vi "Save-Screen-Shot.vi"(11 "VI Path":path) -> (0 "error out":errorcluster)   [LabVIEW 2017]
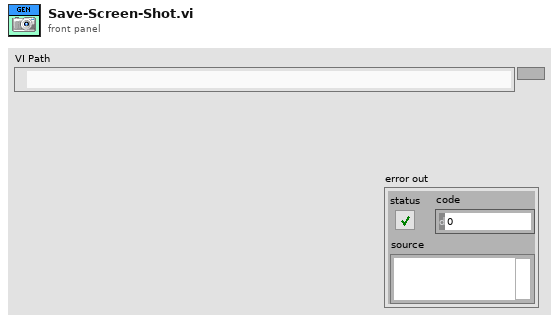
[diagram p1: front panel]
types:
  T1 = typedef "imagedata.ctl" = cluster{"image type":i32, "image depth":i32, "image":u8[], "mask":u8[], "colors":u32[], "Rectangle":cluster{"left":i16, "top":i16, "right":i16, "bottom":i16}}
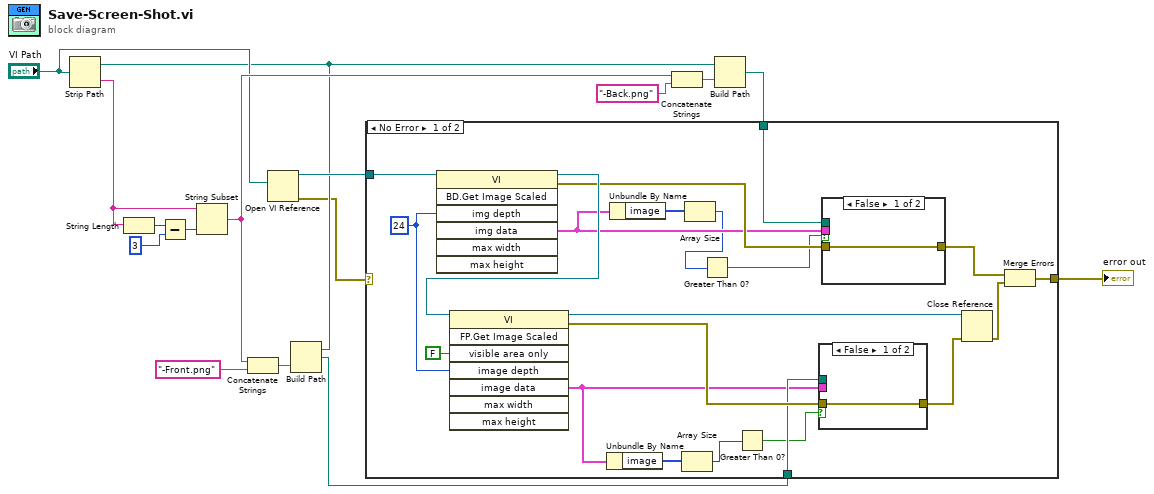
[diagram p0: block diagram]
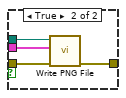
[diagram p2: hidden frame]
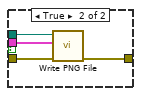
[diagram p3: hidden frame]
diagram:
  n1 = Strip Path(path="VI Path") -> (stripped path=w3:path, name=w2:string)
  n2 = String Length(string=w2) -> (length=w5:i32)
  n3 = Subtract(x=w5, y=3) -> (x-y=w7:i32)
  n4 = String Subset(string=w2, length (rest)=w7) -> (substring=w11:string)  [unwired: 1 in]
  n5 = Concatenate Strings(w11, "-Front.png" ("replace string (\"\")")) -> (w15:string)
  n6 = Open VI Reference(vi path="VI Path") -> (vi reference=w9:refnum<vi>, error out=w1:errorcluster)  [unwired: 5 in]
  n7 = Build Path(base path=w3, name or relative path=w15) -> (appended path=w14:path)
  n8 = Concatenate Strings(w11, "-Back.png" ("replace string (\"\")")) -> (w13:string)
  n9 = Build Path(base path=w3, name or relative path=w13) -> (appended path=w10:path)
  n10 = case shown="No Error" w1 {
    selector: w1 -> [_ w48]
    tunnel: [w33 w48] -> w16
    tunnel: w14 -> [w31 _]
    tunnel: w10 -> [w27 _]
    tunnel: w9 -> [w26 _]
    frame No Error {
      w29 = 24 ("Image Depth")
      n11 = invoke class="VI" method="BD.Get Image Scaled"(reference=w26, "img depth"=w29) -> (reference out=w28:refnum<vi>, error out=w25:errorcluster, "img data"=w24:T1)  [unwired: 5 in, 4 out]
      n12 = invoke class="VI" method="FP.Get Image Scaled"(reference=w28, "visible area only"=FALSE ("Visible Area Only"), "image depth"=w29) -> (reference out=w34:refnum<vi>, error out=w35:errorcluster, "image data"=w19:T1)  [unwired: 5 in, 5 out]
      n13 = Unbundle By Name(w19) -> ("image"=w20:u8[])
      n14 = Unbundle By Name(w24) -> ("image"=w23:u8[])
      n15 = Array Size(array=w20) -> (size(s)=w18:i32)
      n16 = Array Size(array=w23) -> (size(s)=w22:i32)
      n17 = Greater Than 0?(x=w22) -> (x > 0?=w21:bool)
      n18 = Greater Than 0?(x=w18) -> (x > 0?=w17:bool)
      n19 = case shown="False" w17 {
        tunnel: [w38 w42] -> w36
        tunnel: w35 -> [w38 w41]
        tunnel: w31 -> [_ w40]
        tunnel: w19 -> [_ w39]
        frame False {
        }
        frame True {
          n20 = call <vilib>:"Write PNG File.vi"("error in (no error)"=w41, "image data"=w39, "path to PNG file"=w40) -> ("error out"=w42:errorcluster)  [unwired: 7 in, 1 out]
        }
      }
      n21 = case shown="False" w21 {
        tunnel: [w43 w47] -> w32
        tunnel: w27 -> [_ w46]
        tunnel: w25 -> [w43 w45]
        tunnel: w24 -> [_ w44]
        frame False {
        }
        frame True {
          n22 = call <vilib>:"Write PNG File.vi"("error in (no error)"=w45, "image data"=w44, "path to PNG file"=w46) -> ("error out"=w47:errorcluster)  [unwired: 7 in, 1 out]
        }
      }
      n23 = Close Reference(reference=w34, error in (no error)=w36) -> (error out=w37:errorcluster)
      n24 = Merge Errors(w32, w37) -> (w33:errorcluster)
    }
    frame Error {
    }
  }
  "error out" <- w16
